vi "json Insert Boolean - array path.vi"(8 "error in (no error)":errorcluster, 9 "anything":bool, 10 "path":string[](array[string]), 11 "JSON Document in":refnum<class "JSON Document.lvclass">) -> (0 "error out":errorcluster, 1 "replaced?":bool, 3 "JSON Document out":refnum<class "JSON Document.lvclass">)   [LabVIEW 2015, in "JSON Document.lvclass"]
uses:
  JSON Document.lvclass
  json Insert Boolean - string path.vi
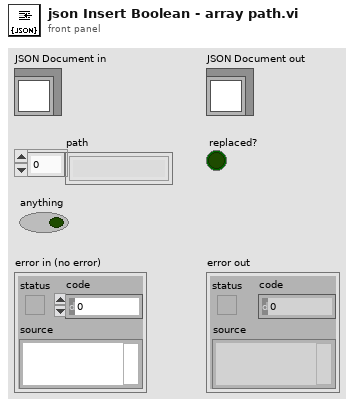
[diagram p1: front panel]
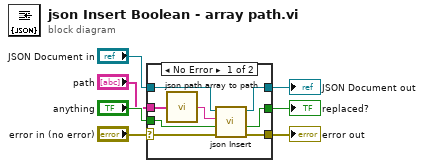
[diagram p0: block diagram]
diagram:
  n1 = case shown="No Error" "error in (no error)" {
    selector: "error in (no error)" -> [w10 w17]
    tunnel: [w9 w17] -> w6
    tunnel: [w14 w16] -> w4
    tunnel: "JSON Document in" -> [w13 w16]
    tunnel: "anything" -> [w11 _]
    tunnel: "path" -> [w15 _]
    tunnel: [w8 _] -> w1
    frame No Error {
      n2 = call "json path array to path.vi"("path"=w15) -> ("String"=w12:string)
      n3 = call-poly "json Insert.vi"("error in (no error)"=w10, "anything"=w11, "path"=w12, "JSON Document in"=w13) -> ("error out"=w9:errorcluster, "replaced?"=w8:bool, "JSON Document out"=w14:refnum<class "JSON Document.lvclass">)  [unwired: 5 in]
    }
    frame Error {
    }
  }
  "error out" <- w6
  "JSON Document out" <- w4
  "replaced?" <- w1
